vi "PiezoSetPosition.vi"(4 "error in (no error)":errorcluster, 5 "lChanID":T1 items=["undefined", "Ch.1", "Ch.2", "Ch.3"], 6 "pos in":sgl min=0 max=20, 7 "reference":refnum<k7>) -> (0 "error out":errorcluster, 3 "reference out":refnum<k7>)   [LabVIEW 2018]
uses:
  <userlib>/bpc203/PiezoChannelNumber.ctl
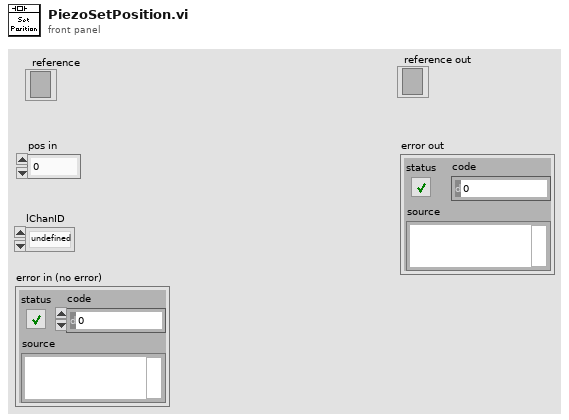
[diagram p1: front panel]
types:
  T1 = typedef "PiezoChannelNumber.ctl" = u16
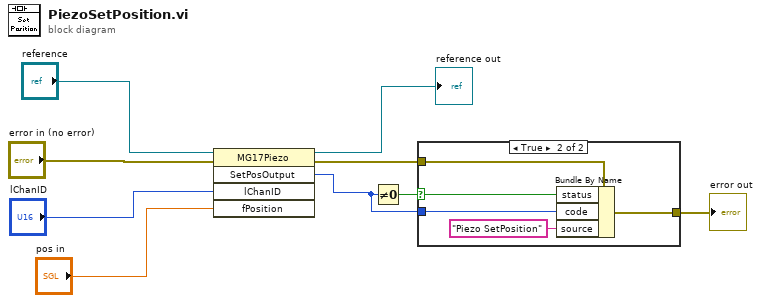
[diagram p0: block diagram]
diagram:
  n1 = invoke class="MG17Piezo" method="SetPosOutput"(reference="reference", error in="error in (no error)", "lChanID"="lChanID", "fPosition"="pos in") -> (reference out=→"reference out":refnum<k7>, error out=w4:errorcluster, "SetPosOutput"=w1:i32)  [unwired: 1 in, 2 out]
  n2 = Not Equal To 0?(x=w1) -> (x != 0?=w5:bool)
  n3 = case shown="True" w5 {
    selector: w5 -> [_ w14]
    tunnel: w4 -> [w10 w15]
    tunnel: [w10 w12] -> w3
    tunnel: w1 -> [_ w11]
    frame False {
    }
    frame True {
      n4 = Bundle By Name(cluster=w15, "status"=w14, "code"=w11, "source"="Piezo SetPosition") -> (w12:errorcluster)
    }
  }
  "error out" <- w3
